vi "Custom Aggregation (Power Symm Comp).vi"(0 "power symmetrical components":T2, 1 "reset? (F)":bool, 5 "aggregation settings":T1={"interval"=1, "interval unit"=enum."Runs", "synchronization of intervals"=enum."Not synchronized", "algorithm"=enum."Average"}, 9 "system info in":refnum<class "EP System Info.lvclass">, 11 "error in (no error)":errorcluster, 12 "data timestamp":timestamp) -> (4 "aggregated minimum value":T2, 6 "aggregated averaged/RMS value":T2, 8 "aggregated maximum value":T2, 10 "system info out":refnum<class "EP System Info.lvclass">, 13 "aggregated data valid?":bool, 14 "aggregated data timestamp":timestamp, 15 "error out":errorcluster)   [LabVIEW 2014, in "NI_EP_Power Quality.lvlib"]
doc: "Calculates the aggregated minimum, maximum, and averaged or RMS value of an input signal for a specified aggregation interval, according to Class S in IEC 61000-4-30:2008. There is no overlap between aggregation intervals. This VI automatically restarts accumulation at the beginning of the next time interval after the previous interval expires. You must manually select the polymorphic instance you want to use.\n\nThis VI supports measuring single-line and multiple-line systems except the DBL instance. Use the DBL instance to measure one channel on one line at one time."
uses:
  <vilib>/addons/Electrical Power/PQ/NI_EP_Power Quality.lvlib
  <vilib>/addons/Electrical Power/PQ/Common/Controls/ep_Aggregation Settings.ctl
  <vilib>/addons/Electrical Power/PQ/Common/Classes/System Info/EP System Info.lvclass
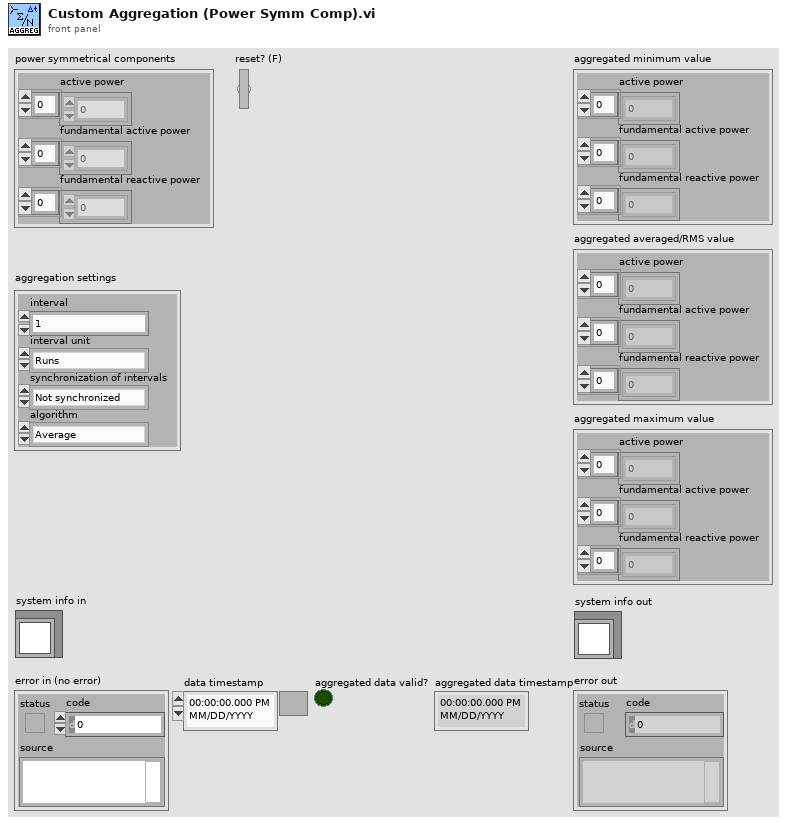
[diagram p1: front panel]
types:
  T1 = typedef "NI_EP_Power Quality.lvlib/ep_Aggregation Settings.ctl" = cluster{"interval":u32, "interval unit":enum16{"Runs", "Seconds", "Minutes", "Hours", "Days", "Weeks"}, "synchronization of intervals":enum16{"Not synchronized", "Interval rounded"}, "algorithm":enum16{"Average", "RMS"}}
  T2 = cluster{"active power":dbl[], "fundamental active power":dbl[], "fundamental reactive power":dbl[]}
  T3 = cluster{"aggregated minimum values":dbl[], "aggregated minimum values":dbl[], "aggregated minimum values":dbl[]}
  T4 = cluster{"aggregated averaged/RMS values":dbl[], "aggregated averaged/RMS values":dbl[], "aggregated averaged/RMS values":dbl[]}
  T5 = cluster{"aggregated maximum values":dbl[], "aggregated maximum values":dbl[], "aggregated maximum values":dbl[]}
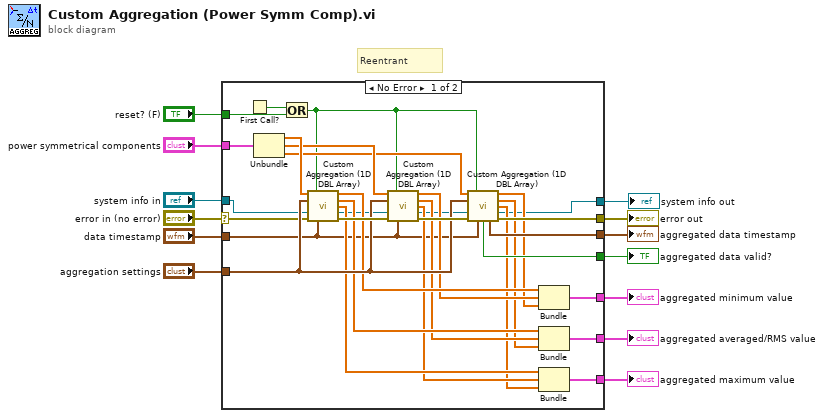
[diagram p0: block diagram]
diagram:
  # "Reentrant"
  n1 = case shown="No Error" "error in (no error)" {
    selector: "error in (no error)" -> [w22 w46]
    tunnel: "reset? (F)" -> [w20 _]
    tunnel: "power symmetrical components" -> [w42 _]
    tunnel: [w41 _] -> w11
    tunnel: [w40 _] -> w10
    tunnel: [w39 _] -> w9
    tunnel: [w38 _] -> w4
    tunnel: [w37 w46] -> w8
    tunnel: "data timestamp" -> [w18 _]
    tunnel: "aggregation settings" -> [w33 _]
    tunnel: [w26 _] -> w3
    tunnel: "system info in" -> [w17 w45]
    tunnel: [w14 w45] -> w1
    frame No Error {
      n2 = First Call?() -> (First Call?: T/F=w21:bool)
      n3 = Unbundle(w42) -> ("active power"=w36:dbl[], "fundamental active power"=w35:dbl[], "fundamental reactive power"=w34:dbl[])
      n4 = Or(x=w21, y=w20) -> (x .or. y?=w19:bool)
      n5 = call <vilib>:"Custom Aggregation (1D DBL Array).vi"("data in"=w36, "reset? (F)"=w19, "aggregation settings"=w33, "system info in"=w17, "error in (no error)"=w22, "data timestamp"=w18) -> ("aggregated minimum values"=w32:dbl[], "aggregated averaged/RMS values"=w31:dbl[], "aggregated maximum values"=w30:dbl[], "system info out"=w16:refnum<class "EP System Info.lvclass">, "error out"=w44:errorcluster)  [unwired: 3 in, 2 out]
      n6 = call <vilib>:"Custom Aggregation (1D DBL Array).vi"("data in"=w35, "reset? (F)"=w19, "aggregation settings"=w33, "system info in"=w16, "error in (no error)"=w44, "data timestamp"=w18) -> ("aggregated minimum values"=w29:dbl[], "aggregated averaged/RMS values"=w28:dbl[], "aggregated maximum values"=w27:dbl[], "system info out"=w15:refnum<class "EP System Info.lvclass">, "error out"=w43:errorcluster)  [unwired: 3 in, 2 out]
      n7 = call <vilib>:"Custom Aggregation (1D DBL Array).vi"("data in"=w34, "reset? (F)"=w19, "aggregation settings"=w33, "system info in"=w15, "error in (no error)"=w43, "data timestamp"=w18) -> ("aggregated minimum values"=w25:dbl[], "aggregated averaged/RMS values"=w24:dbl[], "aggregated maximum values"=w23:dbl[], "system info out"=w14:refnum<class "EP System Info.lvclass">, "aggregated data valid?"=w26:bool, "aggregated data timestamp"=w38:timestamp, "error out"=w37:errorcluster)  [unwired: 3 in]
      n8 = Bundle("aggregated minimum values"=w32, "aggregated minimum values"=w29, "aggregated minimum values"=w25) -> (w41:T3)  [unwired: 1 in]
      n9 = Bundle("aggregated averaged/RMS values"=w31, "aggregated averaged/RMS values"=w28, "aggregated averaged/RMS values"=w24) -> (w40:T4)  [unwired: 1 in]
      n10 = Bundle("aggregated maximum values"=w30, "aggregated maximum values"=w27, "aggregated maximum values"=w23) -> (w39:T5)  [unwired: 1 in]
    }
    frame Error {
    }
  }
  "aggregated minimum value" <- w11
  "aggregated averaged/RMS value" <- w10
  "aggregated maximum value" <- w9
  "error out" <- w8
  "aggregated data valid?" <- w3
  "aggregated data timestamp" <- w4
  "system info out" <- w1
